vi "GetNextPlayer.vi"(11 "current":T1) -> (3 "next":T1)   [LabVIEW 2020]
uses:
  controls/Player.ctl
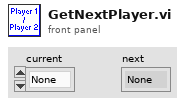
[diagram p1: front panel]
types:
  T1 = typedef "Player.ctl" = enum16{"None", "Player 1", "Player 2"}
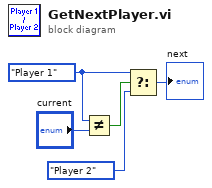
[diagram p0: block diagram]
diagram:
  w4 = Player."Player 1" ("y")
  n1 = Not Equal?(x=w4, y="current") -> (x != y?=w1:bool)
  n2 = Select(t=w4, s=w1, f=Player."Player 2") -> (s? t:f=→"next":T1)
